vi "Ping.vi"(6 "timeout (1000 ms)":i32=1000, 8 "error in (no error)":errorcluster, 11 "Client in":refnum<class "Client.lvclass">) -> (0 "error out":errorcluster, 1 "Server responded":bool, 2 "ping time":i32, 3 "Client out":refnum<class "Client.lvclass">)   [LabVIEW 2013, in "MQTT Client.lvlib" / "Client.lvclass"]
uses:
  Client.lvclass
  <vilib>/LabVIEW Open Source Project/MQTT Control Packets/Control Packets/PINGRESP/PINGRESP.lvclass
  <vilib>/LabVIEW Open Source Project/MQTT Control Packets/Control Packets/PINGREQ/PINGREQ.lvclass
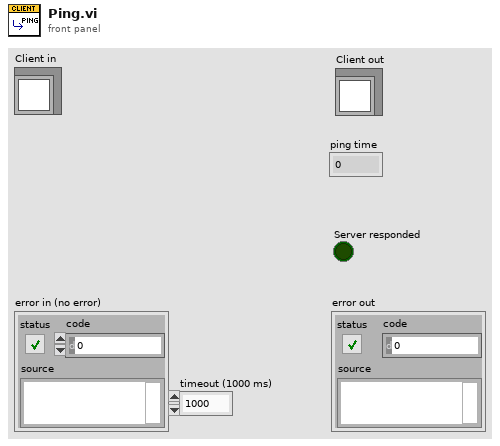
[diagram p1: front panel]
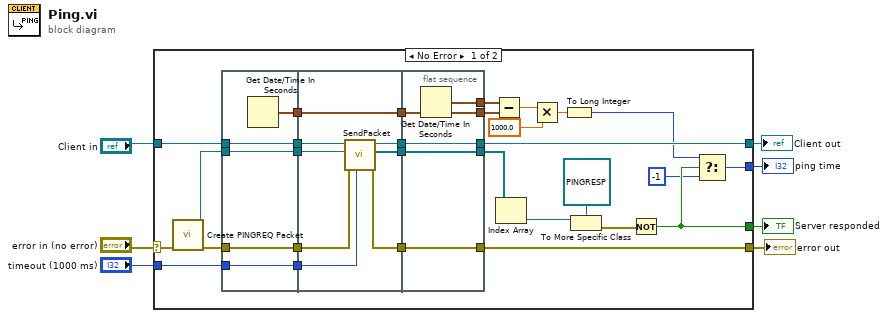
[diagram p0: block diagram]
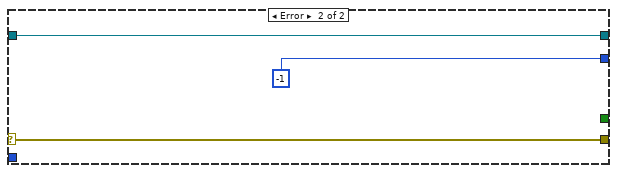
[diagram p2: hidden frame]
diagram:
  n1 = case shown="No Error" "error in (no error)" {
    selector: "error in (no error)" -> [w34 w57]
    tunnel: [w30 w57] -> w4
    tunnel: [w35 w56] -> w5
    tunnel: "Client in" -> [w36 w56]
    tunnel: "timeout (1000 ms)" -> [w32 _]
    tunnel: [w26 _] -> w2
    tunnel: [w25 -1 ("ping time")] -> w1
    frame No Error {
      n2 = call <vilib>:"Create PINGREQ Packet.vi"("error in (no error)"=w34) -> ("error out"=w33:errorcluster, "PINGREQ out"=w23:refnum<class "PINGREQ.lvclass">)  [unwired: 8 in, 1 out]
      n3 = flat-sequence {
        tunnel: w23 -> [w38]
        tunnel: w32 -> [w39]
        tunnel: w33 -> [w40]
        tunnel: w36 -> [w41]
        tunnel: [w41] -> w22
        tunnel: [w40] -> w21
        tunnel: [w39] -> w20
        tunnel: [w38] -> w19
        tunnel: [w37] -> w14
        tunnel: w22 -> [w49]
        tunnel: w21 -> [w47]
        tunnel: w20 -> [w46]
        tunnel: w19 -> [w43]
        tunnel: [w48] -> w18
        tunnel: [w45] -> w17
        tunnel: [w44] -> w16
        tunnel: w14 -> [w42]
        tunnel: [w42] -> w13
        tunnel: [w52] -> w29
        tunnel: [w53] -> w30
        tunnel: [w54] -> w35
        tunnel: w18 -> [w54]
        tunnel: w17 -> [w53]
        tunnel: w16 -> [w52]
        tunnel: [w51] -> w15
        tunnel: w13 -> [w50]
        tunnel: [w50] -> w12
        frame #0 {
          n4 = Get Date/Time In Seconds() -> (seconds since 1Jan1904=w37:timestamp)
        }
        frame #1 {
          n5 = call "SendPacket.vi"("timeout (1000ms)"=w46, "error in (no error)"=w47, "ControlPacket"=w43, "Client in"=w49) -> ("error out"=w45:errorcluster, "Response"=w44:refnum<class "ControlPacket.lvclass">[], "Client out"=w48:refnum<class "Client.lvclass">)  [unwired: 5 in]
        }
        frame #2 {
          n6 = Get Date/Time In Seconds() -> (seconds since 1Jan1904=w51:timestamp)
        }
      }
      n7 = Subtract(x=w15, y=w12) -> (x-y=w11:dbl)
      n8 = Index Array(array=w29) -> (element=w28:refnum<class "ControlPacket.lvclass">)  [unwired: 1 in]
      n9 = Multiply(x=w11, y=1000.0) -> (x*y=w9:dbl)
      n10 = To Long Integer(number=w9) -> (32bit integer=w8:i32)
      n11 = To More Specific Class(target class=refnum<class "PINGRESP.lvclass"> refnum ("PINGRESP.lvclass"), reference=w28) -> (error out=w27:errorcluster)  [unwired: 1 in, 1 out]
      n12 = Not(x=w27) -> (.not. x?=w26:bool)
      n13 = Select(t=w8, s=w26, f=-1 ("ping time")) -> (s? t:f=w25:i32)
    }
    frame Error {
    }
  }
  "error out" <- w4
  "Client out" <- w5
  "Server responded" <- w2
  "ping time" <- w1
